vi "Time to subscribe.vi"(8 "error in (no error)":errorcluster, 11 "Integrate in":refnum<class "Integrate.lvclass">) -> (0 "error out":errorcluster, 3 "Integrate out":refnum<class "Integrate.lvclass">)   [LabVIEW 2015, in "Integrate.lvclass"]
uses:
  Integrate.lvclass
  <vilib>/ActorFramework/Actor/Actor.lvclass/Actor.ctl
  <vilib>/ActorFramework/Message Enqueuer/Message Enqueuer.lvclass/Message Enqueuer.ctl
  Measure_core/Measure Object Messages/Subscribe Request Msg/Subscribe Request Msg.lvclass/Subscribe Request Msg.ctl
  Measure_core/Measure Object/Read Name.vi
  <vilib>/ActorFramework/Message Enqueuer/Init from Existing Queue.vi
  <vilib>/ActorFramework/Message Enqueuer/Enqueue.vi
  <vilib>/ActorFramework/Message Priority Queue/Priority Enqueue.vi
  <vilib>/ActorFramework/Message Enqueuer/Message Enqueuer.lvclass
  Measure_core/Measure Object Messages/Subscribe Request Msg/Subscribe Request Msg.lvclass
  <vilib>/ActorFramework/Actor/Actor.lvclass
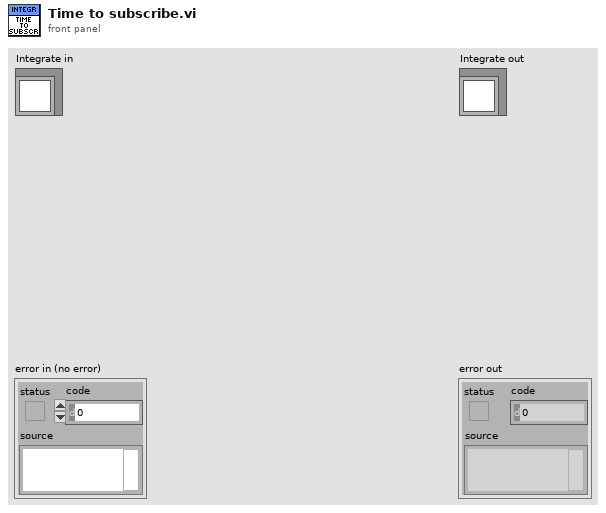
[diagram p1: front panel]
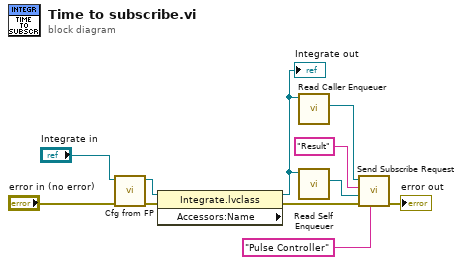
[diagram p0: block diagram]
diagram:
  n1 = call-dynamic "Cfg from FP.vi"("error in (no error)"="error in (no error)", "Measure Object in"="Integrate in") -> ("error out"=w5:errorcluster, "Measure Object out"=w7:refnum<class "Integrate.lvclass">)  [unwired: 8 in]
  n2 = property class="Integrate.lvclass" props=["Accessors:Name"](reference=w7, error in=w5) -> (reference out=w4:refnum<class "Integrate.lvclass">, error out=w10:errorcluster)  [unwired: 1 out]
  "Integrate out" <- w4
  n3 = call <vilib>:"Read Caller Enqueuer.vi"("Actor"=w4) -> ("Caller Enqueuer"=w11:refnum<class "Message Enqueuer.lvclass">)  [unwired: 10 in]
  n4 = call <vilib>:"Read Self Enqueuer.vi"("Actor"=w4) -> ("Self Enqueuer"=w3:refnum<class "Message Enqueuer.lvclass">)  [unwired: 10 in]
  n5 = call "Send Subscribe Request.vi"("Broadcaster"="Pulse Controller" ("Name"), "error in (no error)"=w10, "Subscriber Enqueuer"=w3, "Topic"="Result", "Message Enqueuer"=w11) -> ("error out"=→"error out":errorcluster)  [unwired: 5 in, 1 out]
